vi "LogArm.vi"(8 "Error In":errorcluster, 10 "Setup":T1={"DUT"={"Count"=1, "Wirings"=[], "Names"=[]}, "Log"={"Start"={"Trigger Type"=enum."Immediate", "Timer (sec)"=0.0, "Digital IO Line"=0, "Digital IO Edge"=enum."Rising"}, "Rollover"={"Trigger Type"=enum."None", "Timer (sec)"=0.0, "File Size (MB)"=0, "Digital IO Line"=0, "Digital IO Edge"=enum."Rising"}, "Stop"={"Trigger Type"=enum."None", "Timer (sec)"=0.0, "File Size (MB)"=0, "Digital IO Line"=0, "Digital IO Edge"=enum."Rising"}}, "Trigger"={"Input"={"Type"=enum."None", "Timeout (ms)"=0, "Delay (ms)"=0, "Digital IO Line (1-14)"=0, "Digital IO Mode"=enum."Falling"}, "Output"={"Type"=enum."None", "Delay (ms)"=0, "Digital IO Line (1-14)"=0, "Digital IO Mode"=enum."Falling", "Digital IO Pulse Width (sec)"=0.0}}, "Sources"=[], "Measures"=[]} {"Measures"."Count" min=1 step=1; "Trigger"."Output"."Digital IO Line (1-14)" min=1 max=14 step=1}, 11 "Log Data In":refnum<queue>) -> (0 "Error Out":errorcluster, 3 "Triggered?":bool)   [LabVIEW 2012]
uses:
  Setup.ctl
  DUTConfiguration.ctl
  driver/Public/Controls/SMUSense.ctl
  LogConfiguration.ctl
  LogStartConfiguration.ctl
  LogStartTriggerType.ctl
  LogDigitalIOTriggerEdge.ctl
  LogRolloverConfiguration.ctl
  LogRolloverTriggerType.ctl
  LogStopConfiguration.ctl
  LogStopTriggerType.ctl
  TriggerConfiguration.ctl
  TriggerInputConfiguration.ctl
  TriggerInputType.ctl
  driver/Public/Controls/TriggerMode.ctl
  TriggerOutputConfiguration.ctl
  TriggerOutputType.ctl
  SourceConfiguration.ctl
  SourceFunction.ctl
  MeasureConfiguration.ctl
  HardwareLogData.ctl
  HardwareDisplayData.ctl
  driver/Keithley-2602.lvlib
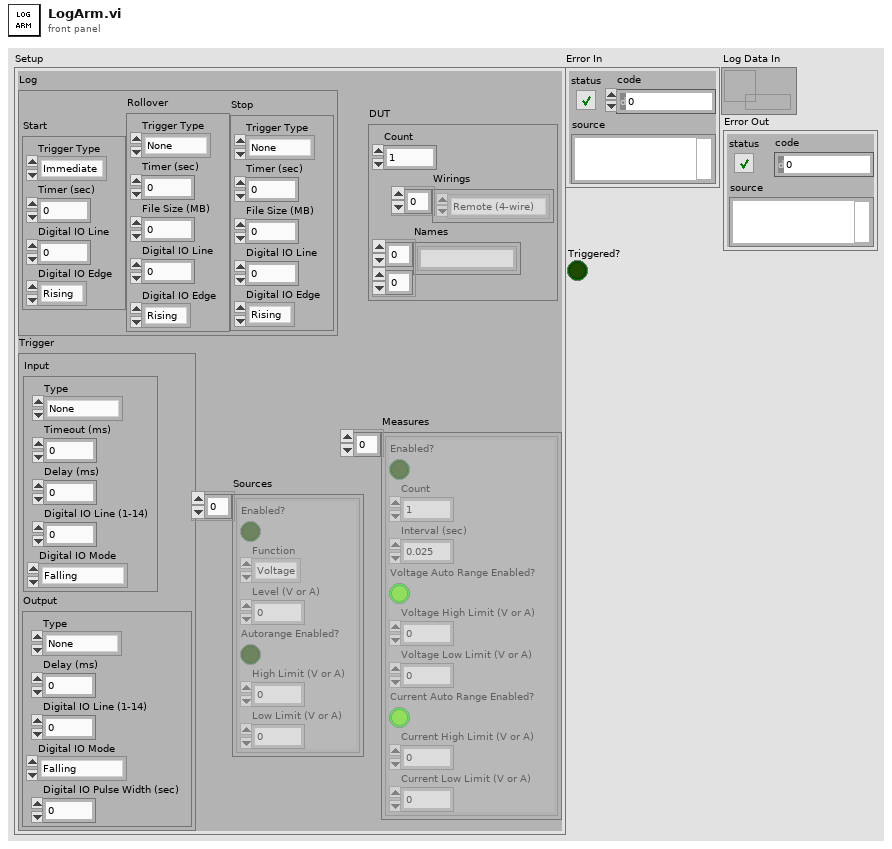
[diagram p1: front panel]
types:
  T1 = typedef "Setup.ctl" = cluster{"DUT":T2, "Log":T4, "Trigger":T12, "Sources":T18[], "Measures":T20[]}
  T2 = typedef "DUTConfiguration.ctl" = cluster{"Count":u32, "Wirings":T3[], "Names":string[][]}
  T3 = typedef "Keithley-2602.lvlib/SMUSense.ctl" = enum16{"Local (2-wire)", "Remote (4-wire)", "Calibration"}
  T4 = typedef "LogConfiguration.ctl" = cluster{"Start":T5, "Rollover":T8, "Stop":T10}
  T5 = typedef "LogStartConfiguration.ctl" = cluster{"Trigger Type":T6, "Timer (sec)":dbl, "Digital IO Line":u8, "Digital IO Edge":T7}
  T6 = typedef "LogStartTriggerType.ctl" = enum16{"Immediate", "User", "Timer", "Digital IO"}
  T7 = typedef "LogDigitalIOTriggerEdge.ctl" = enum16{"Rising", "Falling"}
  T8 = typedef "LogRolloverConfiguration.ctl" = cluster{"Trigger Type":T9, "Timer (sec)":dbl, "File Size (MB)":u32, "Digital IO Line":u8, "Digital IO Edge":T7}
  T9 = typedef "LogRolloverTriggerType.ctl" = enum16{"None", "Timer", "File Size", "Digital IO"}
  T10 = typedef "LogStopConfiguration.ctl" = cluster{"Trigger Type":T11, "Timer (sec)":dbl, "File Size (MB)":u32, "Digital IO Line":u8, "Digital IO Edge":T7}
  T11 = typedef "LogStopTriggerType.ctl" = enum16{"None", "User", "Timer", "File Size", "Digital IO"}
  T12 = typedef "TriggerConfiguration.ctl" = cluster{"Input":T13, "Output":T16}
  T13 = typedef "TriggerInputConfiguration.ctl" = cluster{"Type":T14, "Timeout (ms)":u32, "Delay (ms)":u32, "Digital IO Line (1-14)":u8, "Digital IO Mode":T15}
  T14 = typedef "TriggerInputType.ctl" = enum16{"None", "Digital IO", "Bus"}
  T15 = typedef "Keithley-2602.lvlib/TriggerMode.ctl" = enum16{"Falling", "Rising", "Either", "Synchronous"}
  T16 = typedef "TriggerOutputConfiguration.ctl" = cluster{"Type":T17, "Delay (ms)":u32, "Digital IO Line (1-14)":u8, "Digital IO Mode":T15, "Digital IO Pulse Width (sec)":dbl}
  T17 = typedef "TriggerOutputType.ctl" = enum16{"None", "Digital IO", "Bus"}
  T18 = typedef "SourceConfiguration.ctl" = cluster{"Enabled?":bool, "Function":T19, "Level (V or A)":dbl, "Autorange Enabled?":bool, "High Limit (V or A)":dbl, "Low Limit (V or A)":dbl}
  T19 = typedef "SourceFunction.ctl" = enum16{"Voltage", "Current"}
  T20 = typedef "MeasureConfiguration.ctl" = cluster{"Enabled?":bool, "Count":u8, "Interval (sec)":dbl, "Voltage Auto Range Enabled?":bool, "Voltage High Limit (V or A)":dbl, "Voltage Low Limit (V or A)":dbl, "Current Auto Range Enabled?":bool, "Current High Limit (V or A)":dbl, "Current Low Limit (V or A)":dbl}
  T21 = typedef "HardwareLogData.ctl" = cluster{"Timestamp":timestamp, "Data":T22}
  T22 = typedef "HardwareDisplayData.ctl" = cluster{"DUT Names":string[][], "SMU":dbl[][], "Port":bool[]}
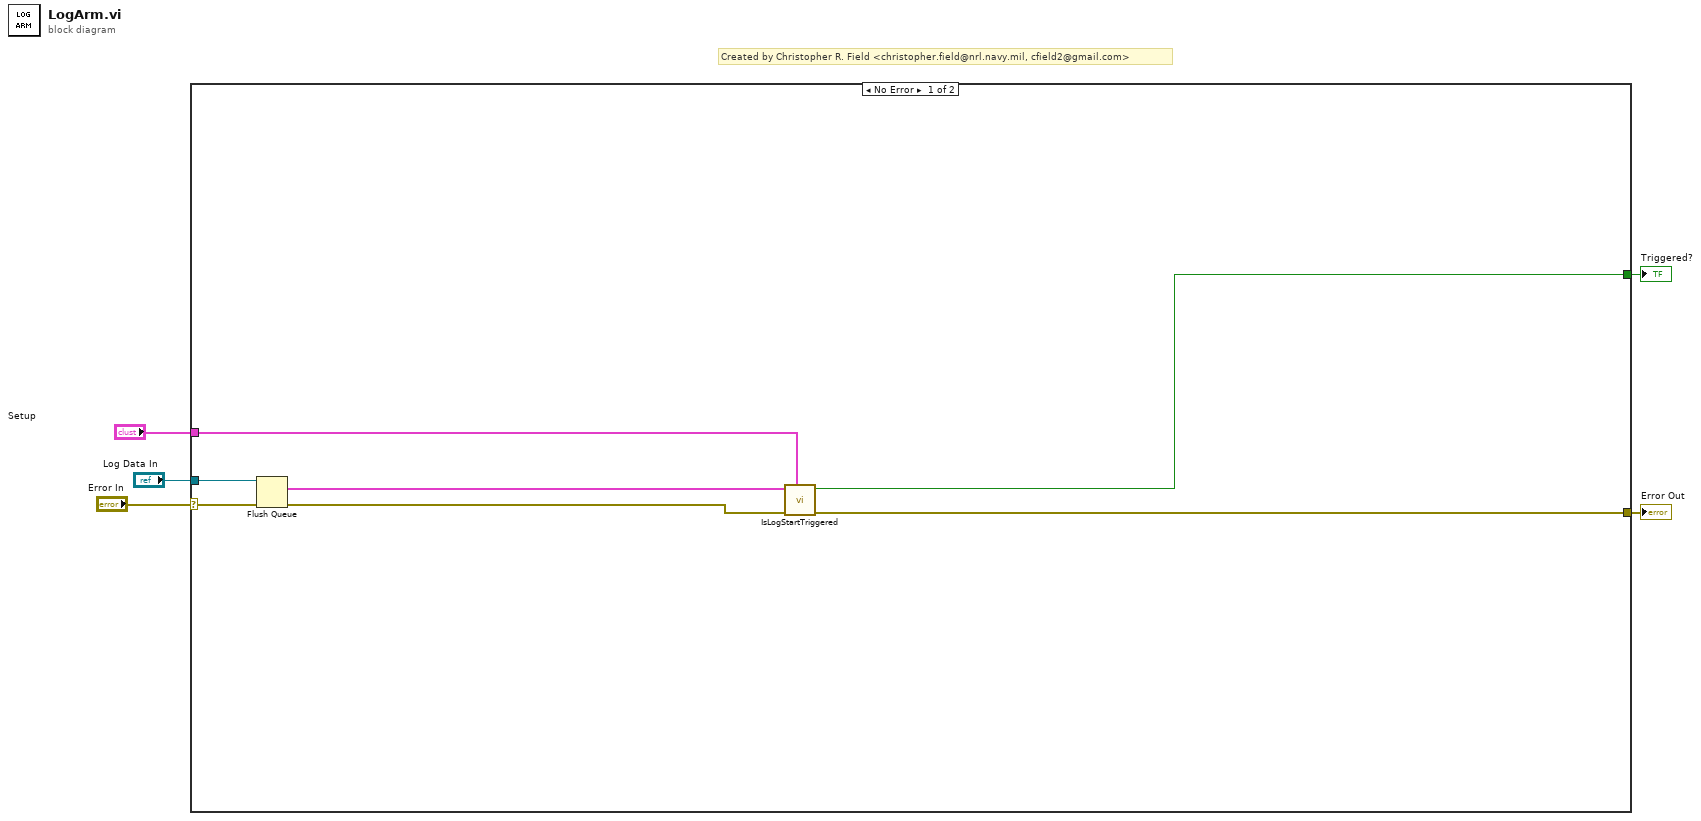
[diagram p0: block diagram]
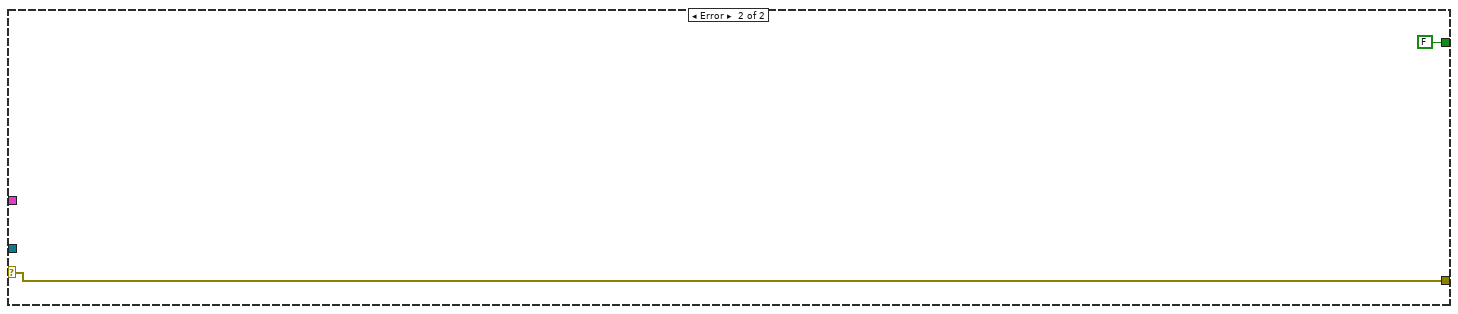
[diagram p2: hidden frame]
diagram:
  # "Created by Christopher R. Field <christopher.field@nrl.navy.mil, cfield2@gmail.com>"
  n1 = case shown="No Error" "Error In" {
    selector: "Error In" -> [w9 w14]
    tunnel: "Setup" -> [w12 _]
    tunnel: "Log Data In" -> [w10 _]
    tunnel: [w6 w14] -> w2
    tunnel: [w11 FALSE ("Triggered?")] -> w1
    frame No Error {
      n2 = Flush Queue(queue=w10, error in (no error)=w9) -> (remaining elements=w8:T21[], error out=w7:errorcluster)  [unwired: 1 out]
      n3 = call "IsLogStartTriggered.vi"("Application Configuration"=w12, "Error In"=w7, "Log Data"=w8) -> ("Error Out"=w6:errorcluster, "Triggered?"=w11:bool)  [unwired: 7 in]
    }
    frame Error {
    }
  }
  "Error Out" <- w2
  "Triggered?" <- w1
